vi "Destroy Logger.vi"(8 "error in (no error)":errorcluster, 11 "Logger in":refnum<class "Logger.lvclass">) -> (0 "error out":errorcluster, 3 "Logger out":refnum<class "Logger.lvclass">)   [LabVIEW 2017, in "Error Log.lvlib" / "Logger.lvclass"]
doc: "Closes all handlers and removes them from the logger."
uses:
  Logger.lvclass
  Logger.lvclass/Logger.ctl
  Get Handlers.vi
  Handler/Handler.lvclass
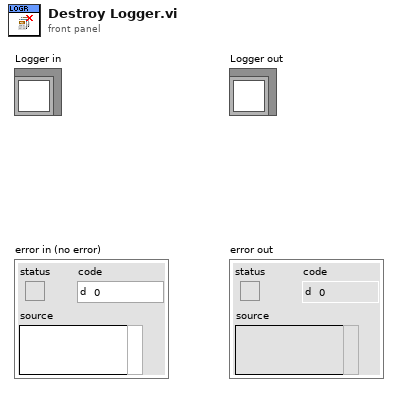
[diagram p1: front panel]
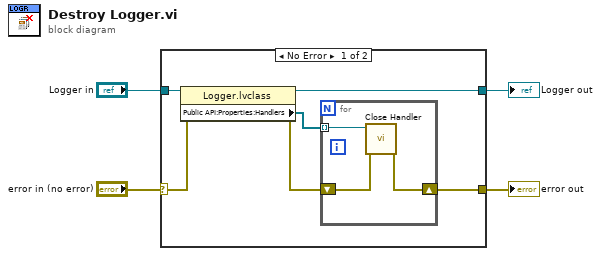
[diagram p0: block diagram]
diagram:
  n1 = case shown="No Error" "error in (no error)" {
    selector: "error in (no error)" -> [w7 w15]
    tunnel: [w9 w15] -> w3
    tunnel: [w8 w14] -> w1
    tunnel: "Logger in" -> [w10 w14]
    frame No Error {
      n2 = property class="Logger.lvclass"(reference=w10, error in=w7) -> (reference out=w8:refnum<class "Logger.lvclass">, error out=w6:errorcluster, "Public API:Properties:Handlers"=w5:refnum<class "Handler.lvclass">[])
      n3 = for {
        tunnel: w5 -> [w13] mode=indexing
        shift-right: [w11] -> w9
        shift-left: w6 -> [w12]
        n4 = call "Close Handler.vi"("error in (no error)"=w12, "Handler in"=w13) -> ("error out"=w11:errorcluster)  [unwired: 8 in, 1 out]
      }
    }
    frame Error {
    }
  }
  "error out" <- w3
  "Logger out" <- w1
